vi "ClearErrorIfWindowDeleted.vi"(7 "Replace Action In":T1=enum."Add or Modify Entry", 8 "error in (no error)":errorcluster, 11 "Window":refnum<class "Window.lvclass">) -> (0 "error out":errorcluster, 5 "Replace Action Out":T1)   [LabVIEW 2020, in "GLF.lvlib" / "Engine.lvclass"]
uses:
  Engine.lvclass
  Engine.lvclass/Engine.ctl
  Window/Window.lvclass
  <vilib>/Utility/miscctls.llb/LVMapReplaceAction.ctl
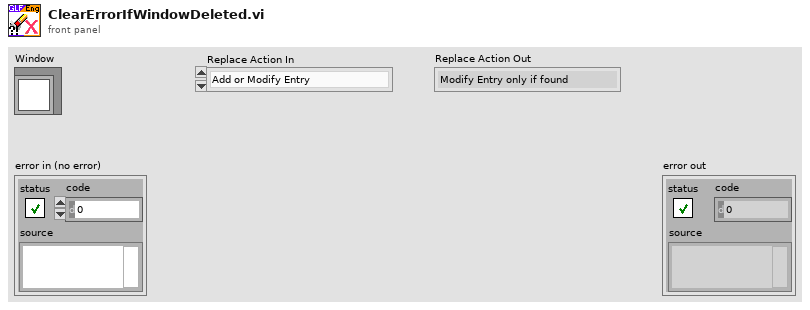
[diagram p1: front panel]
types:
  T1 = typedef "LVMapReplaceAction.ctl" = enum32{"Modify Entry only if found", "Add or Modify Entry", "Delete Entry"}
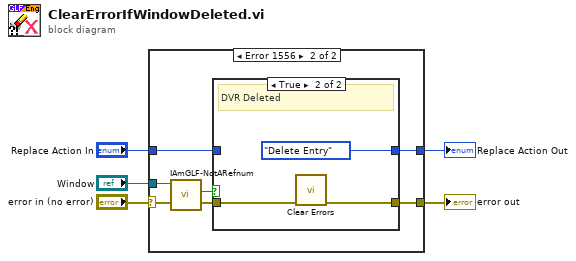
[diagram p0: block diagram]
diagram:
  n1 = case shown="Error 1556" "error in (no error)" {
    selector: "error in (no error)" -> [w7 w13]
    tunnel: [w7 w11] -> w4
    tunnel: "Window" -> [_ w12]
    tunnel: "Replace Action In" -> [w6 w9]
    tunnel: [w6 w8] -> w1
    frame No Error {
      # "Do nothing"
    }
    frame Error {
      n2 = call-dynamic "IAmGLF-NotARefnum.vi"("Window in"=w12) -> ("Not A Valid Refnum?"=w10:bool)  [unwired: 9 in, 1 out]
      n3 = case shown="True" w10 {
        tunnel: w13 -> [w15 w18]
        tunnel: [w15 w17] -> w11
        tunnel: w9 -> [w14 _]
        tunnel: [w14 LVMapReplaceAction."Delete Entry" ("Replace Action In")] -> w8
        frame False {
          # "Other DVR Error"
        }
        frame True {
          # "DVR Deleted"
          n4 = call <vilib>:"Clear Errors.vi"("error in (no error)"=w18) -> ("error out"=w17:errorcluster)  [unwired: 5 in, 1 out]
        }
      }
    }
  }
  "error out" <- w4
  "Replace Action Out" <- w1
